vi "ScalesProperty.vi"(7 "Write?":bool, 8 "error in (no error)":errorcluster, 10 "Values in":sgl[](array[numeric]), 11 "Barcode Detector in":refnum<class "Barcode Detector.lvclass">) -> (0 "error out":errorcluster, 2 "Values out":sgl[](array[numeric]))   [LabVIEW 2020, in "g_ar_toolkit.feature_detection.lvlib" / "Barcode Detector.lvclass"]
uses:
  Barcode Detector.lvclass
  Barcode Detector.lvclass/Barcode Detector.ctl
  g_ar_toolkit.common/g_ar_toolkit.common.lvlib
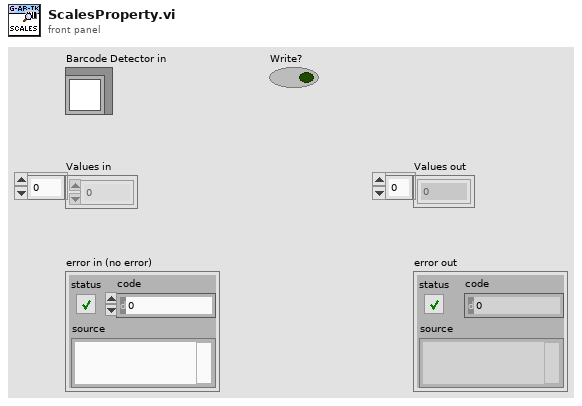
[diagram p1: front panel]
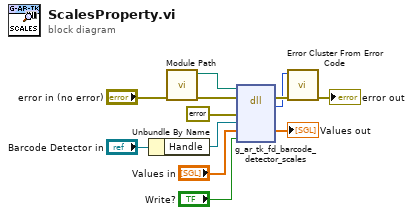
[diagram p0: block diagram]
diagram:
  n1 = Unbundle By Name("Barcode Detector in") -> ("Handle"=w9:refnum<data-value>)
  n2 = call "Module Path.vi"("error in (no error)"="error in (no error)") -> ("error out"=w2:errorcluster, "Path"=w1:path)  [unwired: 9 in]
  n3 = dll-call lib="?" fn="g_ar_tk_fd_barcode_detector_scales" ("g_ar_toolkit.*.*:g_ar_tk_capture_context_create")(path in=w1, error in=w2, "error_cluster"=errorcluster {"status"=FALSE, "code"=0, "source"=""} ("error constant"), "Detector_EDVR"=w9, "Value"="Values in", "Write"="Write?") -> (error out=w6:errorcluster, "MgErr"=w5:i32, "Value"=→"Values out":sgl[])  [unwired: 4 in, 1 out]
  n4 = call <vilib>:"Error Cluster From Error Code.vi"("error in (no error)"=w6, "error code (0)"=w5) -> ("error out"=→"error out":errorcluster)  [unwired: 7 in]
